vi "SendCmd_modbus.vi"(5 "path_bat":path=path "C:/Users/user/Desktop/tool/5.bat", 7 "error in (no error) 2":errorcluster) -> (4 "return code":i32, 6 "Other":string, 8 "release version:":string, 10 "Led Test":string, 14 "error out 3":errorcluster, 15 "version info":string)   [LabVIEW 2017]
panel:
  out "standard output":string
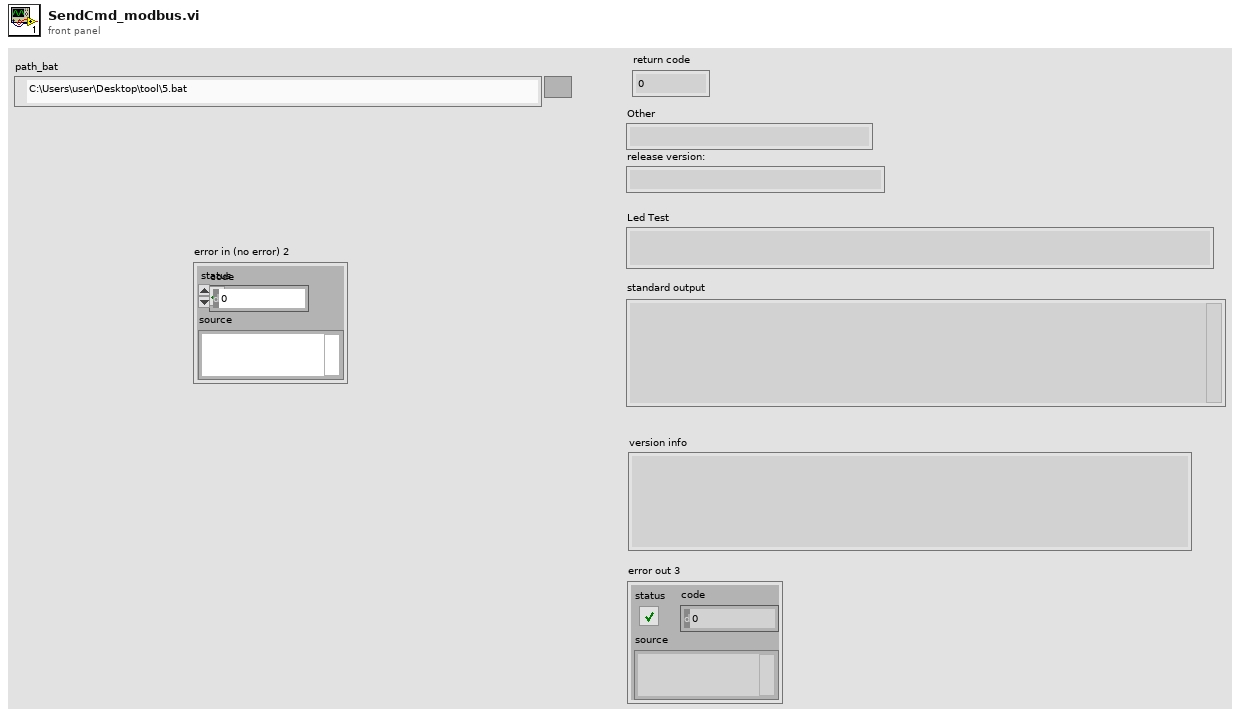
[diagram p1: front panel]
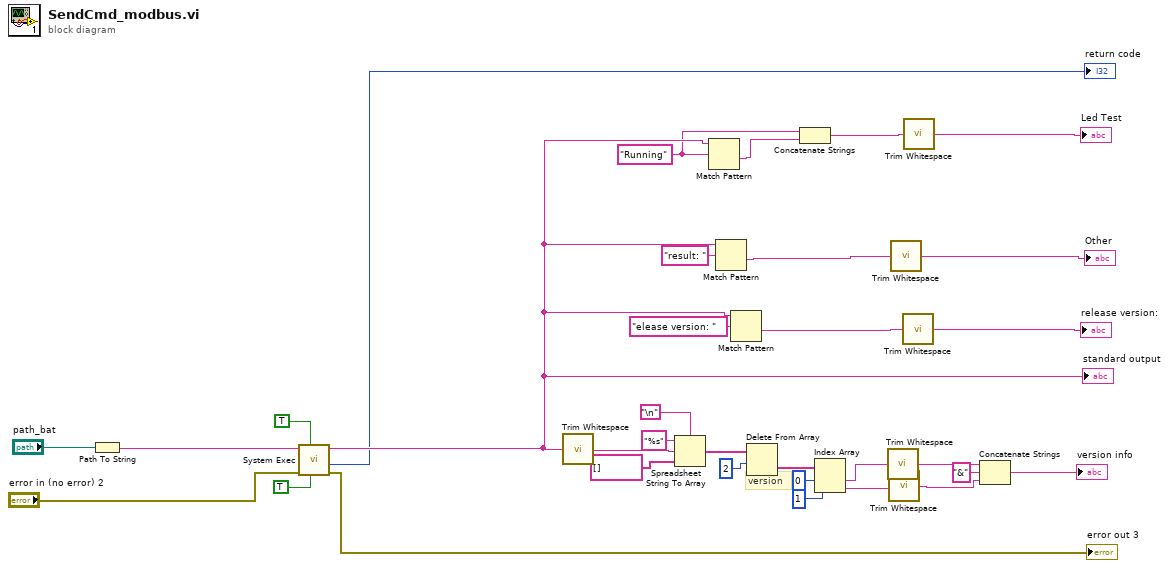
[diagram p0: block diagram]
diagram:
  w8 = "Running" ("regular expression")
  # "version"
  n1 = Path To String(path="path_bat") -> (string=w31:string)
  n2 = call <vilib>:"System Exec.vi"("run minimized? (F)"=TRUE, "wait until completion? (T)"=TRUE, "error in (no error)"="error in (no error) 2", "command line"=w31) -> ("error out"=→"error out 3":errorcluster, "return code"=→"return code":i32, "standard output"=w27:string)  [unwired: 2 in, 3 out]
  "standard output" <- w27
  n3 = call <vilib>:"Trim Whitespace.vi"("string"=w27) -> ("trimmed string"=w22:string)  [unwired: 1 in]
  n4 = Spreadsheet String To Array(delimiter (Tab)="\n", format string="%s", spreadsheet string=w22, array type (2D Dbl)=string[] []) -> (array=w21:string[])
  n5 = Match Pattern(string=w27, regular expression=w8) -> (after substring=w7:string)  [unwired: 1 in, 3 out]
  n6 = Match Pattern(string=w27, regular expression="result: ") -> (after substring=w4:string)  [unwired: 1 in, 3 out]
  n7 = Match Pattern(string=w27, regular expression="elease version: ") -> (after substring=w2:string)  [unwired: 1 in, 3 out]
  n8 = Delete From Array(array=w21, length=2 ("index")) -> (deleted portion=w19:string[])  [unwired: 1 in, 1 out]
  n9 = Concatenate Strings(w8, w7) -> (w6:string)
  n10 = Index Array(array=w19, index #1=0 ("index"), index #2=1 ("index")) -> (element #1=w14:string, element #2=w12:string)
  n11 = call <vilib>:"Trim Whitespace.vi"("string"=w14) -> ("trimmed string"=w13:string)  [unwired: 1 in]
  n12 = call <vilib>:"Trim Whitespace.vi"("string"=w12) -> ("trimmed string"=w11:string)  [unwired: 1 in]
  n13 = call <vilib>:"Trim Whitespace.vi"("string"=w4) -> ("trimmed string"=→"Other":string)  [unwired: 1 in]
  n14 = call <vilib>:"Trim Whitespace.vi"("string"=w2) -> ("trimmed string"=→"release version:":string)  [unwired: 1 in]
  n15 = call <vilib>:"Trim Whitespace.vi"("string"=w6) -> ("trimmed string"=→"Led Test":string)  [unwired: 1 in]
  n16 = Concatenate Strings(w13, "&" ("string"), w11) -> (→"version info":string)
